vi "SwitchBoard_close.vi"(8 "error in":errorcluster, 11 "Handle":u32) -> (0 "error out":errorcluster, 3 "Handle":u32)   [LabVIEW 2016]
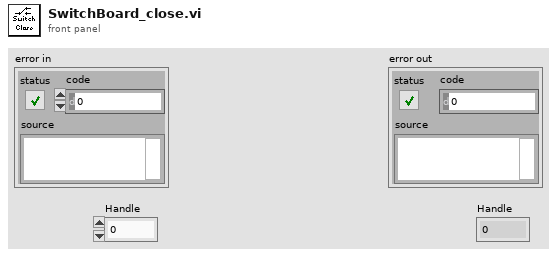
[diagram p1: front panel]
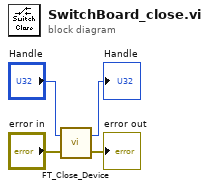
[diagram p0: block diagram]
diagram:
  n1 = call "FT_Close_Device.vi"("error in"="error in", "Handle"="Handle") -> ("error out"=→"error out":errorcluster, "Handle out"=→"Handle":u32)
